vi "CreateTimestampFileName.vi"(10 "File Extension (.csv)":string=".csv", 11 "Time Stamp":timestamp) -> (3 "Timestamp File Name":string)   [LabVIEW 2012, in "LV-Utilities.lvlib"]
uses:
  LV-Utilities.lvlib
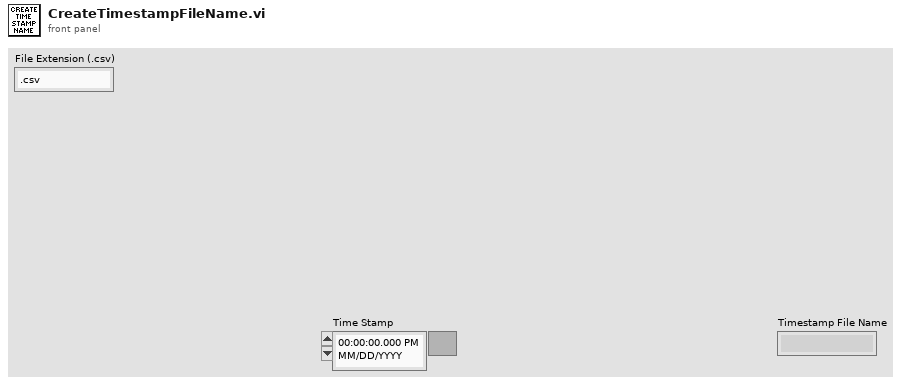
[diagram p1: front panel]
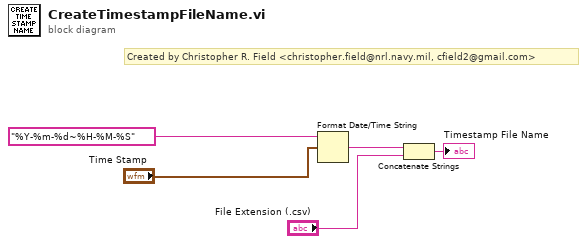
[diagram p0: block diagram]
diagram:
  # "Created by Christopher R. Field <christopher.field@nrl.navy.mil, cfield2@gmail.com>"
  n1 = Format Date/Time String(time format string (%c)="%Y-%m-%d~%H-%M-%S", seconds (now)="Time Stamp") -> (date/time string=w4:string)  [unwired: 1 in]
  n2 = Concatenate Strings(w4, "File Extension (.csv)") -> (→"Timestamp File Name":string)
